vi "Setup.vi"(1 "timeout ms (10000)":i32=10000, 2 "local port (0)":u16, 3 "Remote Port (502)":u16=502, 4 "slave host":string) -> (0 "Modbus TCP Micro Master out":refnum<class "Modbus TCP Micro Master.lvclass">)   [LabVIEW 2023, in "Modbus TCP Micro.lvlib" / "Modbus TCP Micro Master.lvclass"]
uses:
  Modbus TCP Micro Master.lvclass
  Modbus TCP Micro Master.lvclass/Modbus TCP Micro Master.ctl
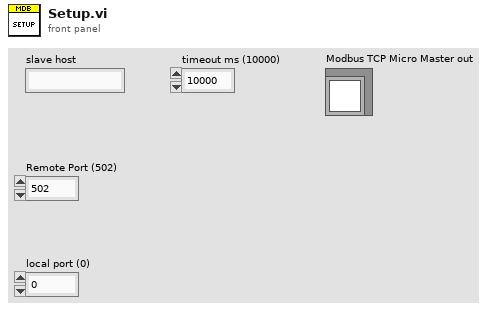
[diagram p1: front panel]
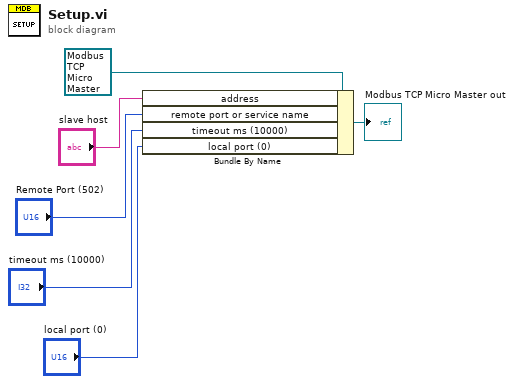
[diagram p0: block diagram]
diagram:
  n1 = Bundle By Name(cluster=refnum<class "Modbus TCP Micro Master.lvclass"> refnum ("Modbus TCP Micro Master in"), "address"="slave host", "remote port or service name"="Remote Port (502)", "timeout ms (10000)"="timeout ms (10000)", "local port (0)"="local port (0)") -> (→"Modbus TCP Micro Master out":refnum<class "Modbus TCP Micro Master.lvclass">)
